vi "Pauli-X_s.vi"(2 "v Ctrl in":refnum<class "CtrlLine.lvclass">[](array[class]), 7 "QuWire in":refnum<class "QuWire.lvclass">, 13 "^ Ctrl in":refnum<class "CtrlLine.lvclass">[](array[class])) -> (8 "QuWire out":refnum<class "QuWire.lvclass">)   [LabVIEW 2020]
doc: "Pauli-X Gate\n\nApplies a bit-flip (NOT). \nMaps |0> to |1> and |1> to |0>. \nRotates by pi radians around the X-axis.\n \nMatrix: [[ 0, 1], [ 1, 0]]"
uses:
  QuSim/QuWire/QuWire.lvclass
  QuSim/QuWire/CtrlLine/CtrlLine.lvclass
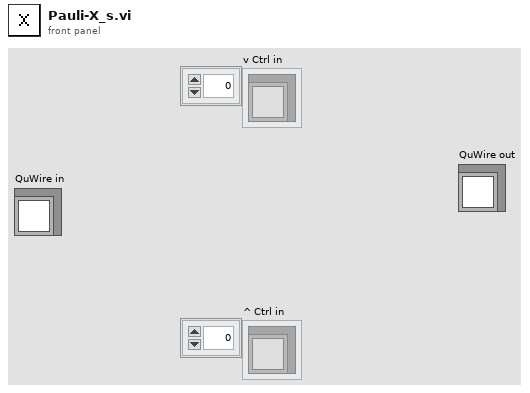
[diagram p1: front panel]
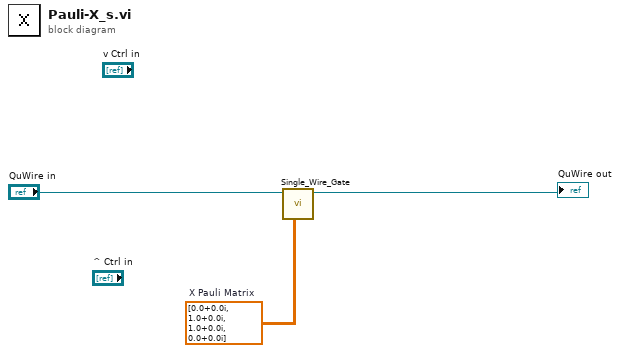
[diagram p0: block diagram]
diagram:
  w1 = cdb[][] [[0.0+0.0i, 1.0+0.0i], [1.0+0.0i, 0.0+0.0i]]  # X Pauli Matrix
  n1 = call "Single_Wire_Gate.vi"("2x2 Unitary Matrix"=w1, "QuWire in"="QuWire in") -> ("QuWire out"=→"QuWire out":refnum<class "QuWire.lvclass">)  [unwired: 8 in, 1 out]
